vi "decodeFeedback.vi"(8 "error in (no error)":errorcluster, 10 "String":string, 11 "Communication in":refnum<class "Communication.lvclass">) -> (0 "error out":errorcluster, 2 "FeedbackData":T1, 3 "Communication out":refnum<class "Communication.lvclass">)   [LabVIEW 2023, in "Communication.lvclass"]
uses:
  Communication.lvclass
  feedbackData.ctl
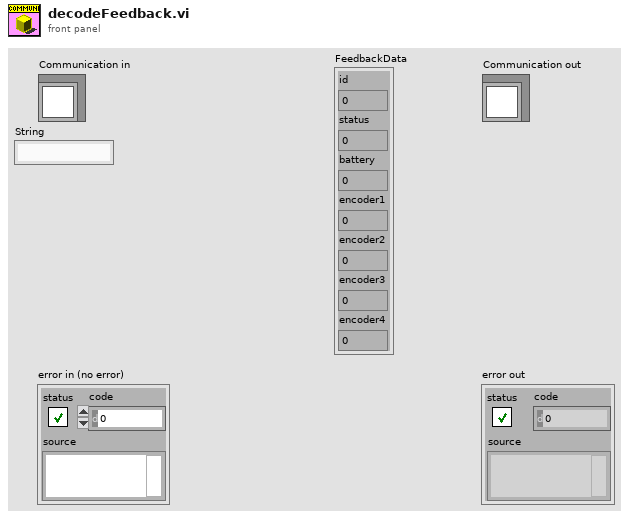
[diagram p1: front panel]
types:
  T1 = typedef "feedbackData.ctl" = cluster{"id":u32, "status":u32, "battery":sgl, "encoder1":sgl, "encoder2":sgl, "encoder3":sgl, "encoder4":sgl}
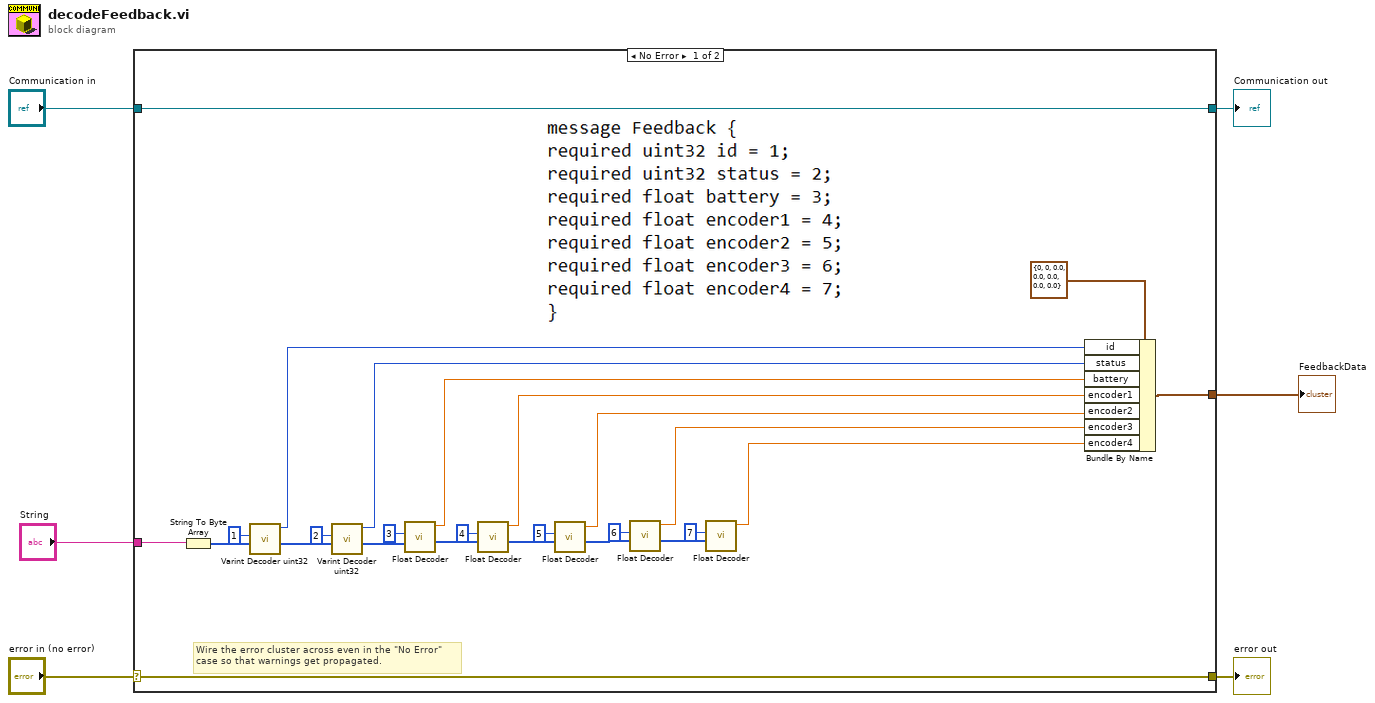
[diagram p0: block diagram]
diagram:
  n1 = case shown="No Error" "error in (no error)" {
    selector: "error in (no error)" -> [w31 w34]
    tunnel: [w31 w34] -> w5
    tunnel: [w32 w33] -> w3
    tunnel: "Communication in" -> [w32 w33]
    tunnel: "String" -> [w30 _]
    tunnel: [w26 _] -> w1
    frame No Error {
      # "Wire the error cluster across even in the \"No Error\"\ncase so that warnings get propagated."
      n2 = String To Byte Array(string=w30) -> (unsigned byte array=w29:u8[])
      n3 = call "Varint Decoder uint32.vi"("Array"=w29, "Key"=1) -> ("array w/ subset deleted"=w25:u8[], "Varint"=w13:u32)  [unwired: 6 in, 2 out]
      n4 = call "Varint Decoder uint32.vi"("Array"=w25, "Key"=2) -> ("array w/ subset deleted"=w23:u8[], "Varint"=w12:u32)  [unwired: 6 in, 2 out]
      n5 = call "Float Decoder.vi"("Array"=w23, "Key"=3) -> ("array w/ subset deleted"=w22:u8[], "Float"=w11:sgl)  [unwired: 6 in, 2 out]
      n6 = call "Float Decoder.vi"("Array"=w22, "Key"=4) -> ("array w/ subset deleted"=w21:u8[], "Float"=w10:sgl)  [unwired: 6 in, 2 out]
      n7 = call "Float Decoder.vi"("Array"=w21, "Key"=5) -> ("array w/ subset deleted"=w20:u8[], "Float"=w9:sgl)  [unwired: 6 in, 2 out]
      n8 = call "Float Decoder.vi"("Array"=w20, "Key"=6) -> ("array w/ subset deleted"=w19:u8[], "Float"=w8:sgl)  [unwired: 6 in, 2 out]
      n9 = call "Float Decoder.vi"("Array"=w19, "Key"=7) -> ("Float"=w7:sgl)  [unwired: 6 in, 3 out]
      n10 = Bundle By Name(cluster=T1 {"id"=0, "status"=0, "battery"=0.0, "encoder1"=0.0, "encoder2"=0.0, "encoder3"=0.0, "encoder4"=0.0} ("FeedbackData"), "id"=w13, "status"=w12, "battery"=w11, "encoder1"=w10, "encoder2"=w9, "encoder3"=w8, "encoder4"=w7) -> (w26:T1)
    }
    frame Error {
    }
  }
  "error out" <- w5
  "Communication out" <- w3
  "FeedbackData" <- w1
